vi "Template Path.vi"(8 "error in":errorcluster, 10 "Template Path":path) -> (0 "error out":errorcluster)   [LabVIEW 2020, in "Data Type Scripting.lvlib"]
doc: "_____\nCreated using DQMH Event Scripter 6.0.0.122."
uses:
  Data Type Scripting.lvlib
  Template Path Argument--cluster.ctl
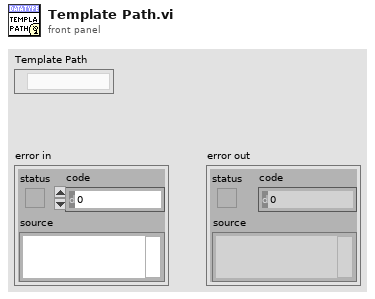
[diagram p1: front panel]
types:
  T1 = typedef "Data Type Scripting.lvlib/Template Path Argument--cluster.ctl" = cluster{"Template Path":path, "Exists?":bool}
  T2 = typedef "Data Type Scripting.lvlib/Broadcast Events--cluster.ctl" = cluster{"Module Did Init":refnum<user-event>, "Status Updated":refnum<user-event>, "Error Reported":refnum<user-event>, "Module Did Stop":refnum<user-event>, "Update Module Execution Status":refnum<user-event>, "Template Path":refnum<user-event>, "Poly List":refnum<user-event>, "Poly Details":refnum<user-event>, "Data Type Valid":refnum<user-event>, "List of Data Types":refnum<user-event>}
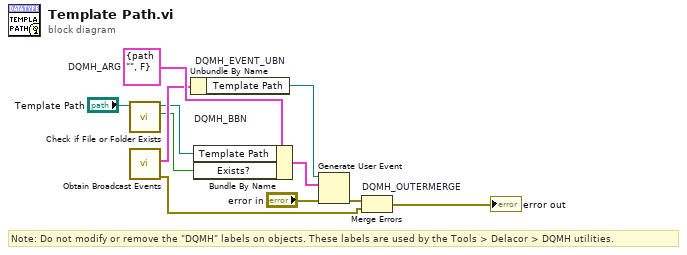
[diagram p0: block diagram]
diagram:
  w6 = T1 {"Template Path"=path "", "Exists?"=FALSE}  # DQMH_ARG
  # "Note: Do not modify or remove the \"DQMH\" labels on objects. These labels are used by the Tools > Delacor > DQMH utilities."
  n1 = call <vilib>:"Check if File or Folder Exists.vi"("path"="Template Path") -> ("file or folder exists?"=w1:bool, "dup path"=w2:path)  [unwired: 8 in, 1 out]
  n2 = call "Obtain Broadcast Events.vi"() -> ("error out"=w5:errorcluster, "Data Type Scripting Broadcast Events"=w4:T2)  [unwired: 10 in]
  n3 = Unbundle By Name "DQMH_EVENT_UBN"(w4) -> ("Template Path"=w8:refnum<user-event>)
  n4 = Bundle By Name "DQMH_BBN"(cluster=w6, "Template Path"=w2, "Exists?"=w1) -> (w9:T1)
  n5 = Generate User Event(user event=w8, event data cluster=w9, error in="error in") -> (error out=w7:errorcluster)  [unwired: 1 in, 1 out]
  n6 = Merge Errors "DQMH_OUTERMERGE"(w7, w5) -> (→"error out":errorcluster)
